vi "Launch Nested Panel.vi"(4 "Auto-stop? (T)":bool=TRUE, 6 "timeout in ms (-1)":i32=-1, 8 "error in (no error)":errorcluster, 9 "Panel":refnum<class "Panel.lvclass">, 10 "Nested Panel Actor":refnum<class "Panel Actor.lvclass">, 11 "Panel Actor in":refnum<class "Panel Actor.lvclass">) -> (0 "error out":errorcluster, 1 "timed out?":bool, 2 "Nested Actor's Enqueuer":refnum<class "Message Enqueuer.lvclass">, 3 "Panel Actor out":refnum<class "Panel Actor.lvclass">)   [LabVIEW 2023, in "Panel Actor.lvlib" / "Panel Actor.lvclass"]
doc: "Launches a new nested Panel Actor with the specified Panel Type.\n\n<B>Panel Actor In:</B> Caller Panel Actor object\n<B>Nested Panel Actor:</B> Panel actor to launch as a nested actor.\n<B>Panel:</B> Panel object for displaying the nested Panel Actor.\n<B>timeout in ms (-1):</B> Sets the timeout for launching the nested actor\n<B>Auto-Stop?:</B> Defines if the actor should stop automatically.\n<B>Error In:</B> Describes error conditions that occur before this node runs.\n\n<B>Panel Actor Out:</B> Caller Panel Actor object.\n<B>timed out?</B> Indicates if the action timed out.\n<B>Error Out:</B> Contains error information.\n----\nPlease see the following web address for additional documentation and tutorial information:\nhttp://www.mooregoodideas.com/mgi-panel-manager/\n\nAuthor: Derek Trepanier\n\nCopyright (c) 2018, Moore Good Ideas, Inc.\n\nAll rights reserved.\n\nRedistribution and use in source and binary forms, with or without modification, are permitted provided that the following conditions are met:\n\n * Redistributions of source code must retain the above copyright notice, this list of conditions and the following disclaimer.\n * Redistributions in binary form must reproduce the above copyright notice, this list of conditions and the following disclaimer in the documentation and/or other materials provided with the distribution.\n * Neither the name of Moore Good Ideas, Inc. nor the names of its contributors may be used to endorse or promote products derived from this software without specific prior written permission.\n\nTHIS SOFTWARE IS PROVIDED BY THE COPYRIGHT HOLDERS AND CONTRIBUTORS \"AS IS\" AND ANY EXPRESS OR IMPLIED WARRANTIES, INCLUDING, BUT NOT LIMITED TO, THE IMPLIED WARRANTIES OF MERCHANTABILITY AND FITNESS FOR A PARTICULAR PURPOSE ARE DISCLAIMED. IN NO EVENT SHALL THE COPYRIGHT OWNER OR CONTRIBUTORS BE LIABLE FOR ANY DIRECT, INDIRECT, INCIDENTAL, SPECIAL, EXEMPLARY, OR CONSEQUENTIAL DAMAGES (INCLUDING, BUT NOT LIMITED TO, PROCUREMENT OF SUBSTITUTE GOODS OR SERVICES; LOSS OF USE, DATA, OR PROFITS; OR BUSINESS INTERRUPTION) HOWEVER CAUSED AND ON ANY THEORY OF LIABILITY, WHETHER IN CONTRACT, STRICT LIABILITY, OR TORT (INCLUDING NEGLIGENCE OR OTHERWISE) ARISING IN ANY WAY OUT OF THE USE OF THIS SOFTWARE, EVEN IF ADVISED OF THE POSSIBILITY OF SUCH DAMAGE."
uses:
  Library/Panel Actor.lvclass
  Panel/Panel/Panel.lvclass
  builds/Framework/Actor Framework.lvlibp/1abvi3w/vi.lib/ActorFramework/Message Enqueuer/Message Enqueuer.lvclass
  Panel/Panel/Panel.lvclass/Panel.ctl
  Library/Panel Actor.lvclass/Panel Actor.ctl
  Panel/Init Waiter/Init Waiter.vi
  Panel/Init Waiter/Init Waiter.lvclass
  builds/Framework/Actor Framework.lvlibp/1abvi3w/vi.lib/ActorFramework/Actor/Actor.lvclass
  C:/Users/Public/Documents/Development/builds/Framework/Actor Framework.lvlibp/1abvi3w/vi.lib/ActorFramework/Actor/Actor.lvclass
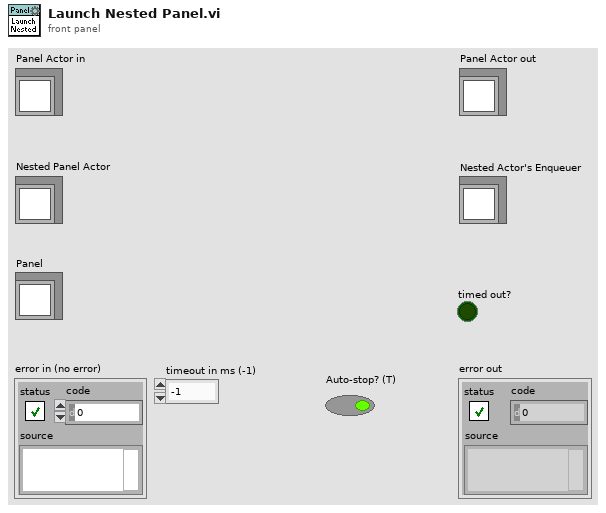
[diagram p1: front panel]
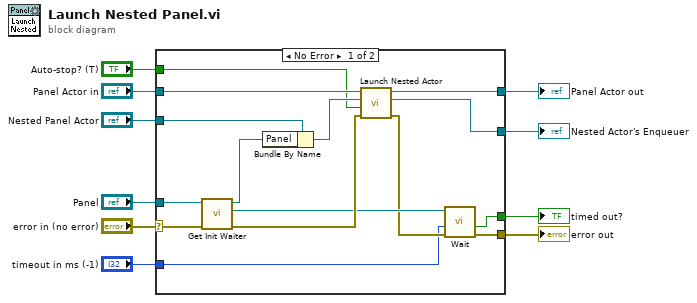
[diagram p0: block diagram]
diagram:
  n1 = case shown="No Error" "error in (no error)" {
    selector: "error in (no error)" -> [w18 w27]
    tunnel: [w15 w27] -> w9
    tunnel: [w23 w26] -> w7
    tunnel: "Panel Actor in" -> [w24 w26]
    tunnel: "Nested Panel Actor" -> [w25 _]
    tunnel: [w21 _] -> w4
    tunnel: "Panel" -> [w19 _]
    tunnel: "Auto-stop? (T)" -> [w20 _]
    tunnel: "timeout in ms (-1)" -> [w13 _]
    tunnel: [w12 _] -> w1
    frame No Error {
      n2 = call "Get Init Waiter.vi"("Error In"=w18, "Panel In"=w19) -> ("Error Out"=w17:errorcluster, "Init Waiter"=w16:refnum<class "Init Waiter.lvclass">, "Panel Out"=w11:refnum<class "Panel.lvclass">)  [unwired: 7 in]
      n3 = Bundle By Name(cluster=w25, "Panel"=w11) -> (w22:refnum<class "Panel Actor.lvclass">)
      n4 = call "Launch Nested Actor.vi"("error in (no error)"=w17, "Auto-stop? (T)"=w20, "Nested Actor"=w22, "Caller Actor in"=w24) -> ("error out"=w14:errorcluster, "Nested Actor's Enqueuer"=w21:refnum<class "Message Enqueuer.lvclass">, "Caller Actor out"=w23:refnum<class "Panel Actor.lvclass">)  [unwired: 5 in]
      n5 = call "Wait.vi"("Error In"=w14, "timeout in ms (-1)"=w13, "Init Waiter in"=w16) -> ("Error Out"=w15:errorcluster, "timed out?"=w12:bool)  [unwired: 7 in]
    }
    frame Error {
    }
  }
  "error out" <- w9
  "Panel Actor out" <- w7
  "Nested Actor's Enqueuer" <- w4
  "timed out?" <- w1
